vi "Write OUR_Monitor.vi"(8 "error in (no error)":errorcluster, 10 "MBPOnOff_Controller.lvlib:OUR_Monitor.lvclass":refnum<class "OUR_Monitor.lvclass">, 11 "Model_Predictor in":refnum<class "Model_Predictor.lvclass">) -> (0 "error out":errorcluster, 3 "Model_Predictor out":refnum<class "Model_Predictor.lvclass">)   [LabVIEW 2021, in "MBPOnOff_Controller.lvlib" / "Model_Predictor.lvclass"]
uses:
  Model_Predictor.lvclass
  OUR_Monitor/OUR_Monitor.lvclass
  Model_Predictor.lvclass/Model_Predictor.ctl
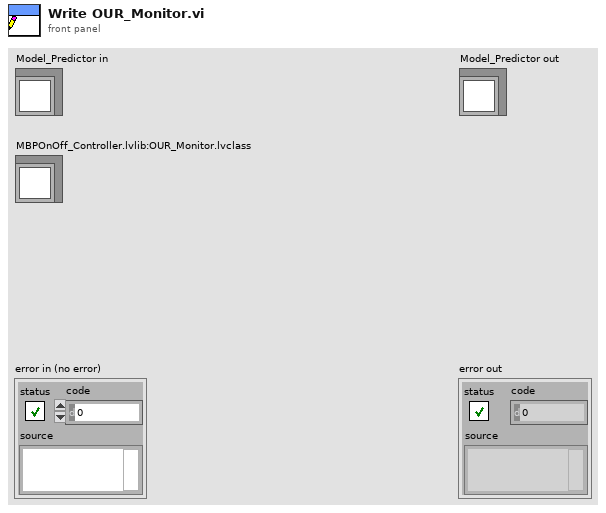
[diagram p1: front panel]
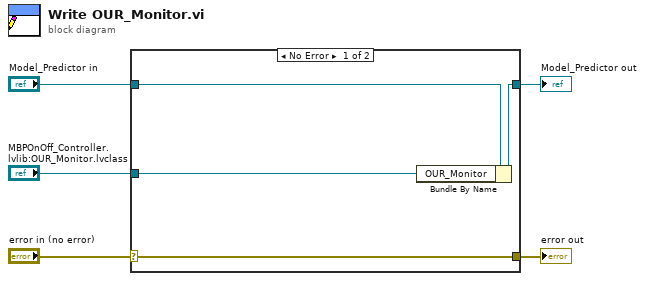
[diagram p0: block diagram]
diagram:
  n1 = case shown="No Error" "error in (no error)" {
    selector: "error in (no error)" -> [w9 w10]
    tunnel: [w9 w10] -> w4
    tunnel: [w7 w11] -> w2
    tunnel: "Model_Predictor in" -> [w8 w11]
    tunnel: "MBPOnOff_Controller.lvlib:OUR_Monitor.lvclass" -> [w6 _]
    frame No Error {
      n2 = Bundle By Name(cluster=w8, "OUR_Monitor"=w6) -> (w7:refnum<class "Model_Predictor.lvclass">)
    }
    frame Error {
    }
  }
  "error out" <- w4
  "Model_Predictor out" <- w2
